vi "HFRR ADV v023 new software.vi"() -> ()   [LabVIEW 2025] (continued)
        n1928 = Divide(x=1705.984, y=w2075) -> (x/y=w2076:dbl)
        n1929 = Divide(x=1705.984, y=w2088) -> (x/y=w2089:dbl)
        n1930 = local read "Humidity before test"() -> (w2080:dbl)
        n1931 = local read "Humidity after test"() -> (w2093:dbl)
        n1932 = Subtract(x=8.017352 ("y"), y=w2076) -> (x-y=w2102:dbl)
        n1933 = Subtract(x=8.017352 ("y"), y=w2089) -> (x-y=w2096:dbl)
        n1934 = expression code="10**y"(w2102) -> (w2082:dbl)
        n1935 = expression code="10**y"(w2096) -> (w2095:dbl)
        n1936 = Multiply(x=w2080, y=w2082) -> (x*y=w2081:dbl)
        n1937 = Multiply(x=w2093, y=w2095) -> (x*y=w2094:dbl)
        n1938 = Divide(x=w2081, y=750.0) -> (x/y=w2097:dbl)
        n1939 = Divide(x=w2094, y=750.0) -> (x/y=w2098:dbl)
        n1940 = Add(x=w2097, y=w2098) -> (x+y=w2099:dbl)
        n1941 = Divide(x=w2099, y=2.0) -> (x/y=w2101:dbl)
        n1942 = local write "AVP"(w2101) -> ()
        n1943 = Subtract(x=1.4, y=w2101) -> (x-y=w2084:dbl)
        n1944 = local read "HCF"() -> (w2085:dbl)
      }
      frame Enabled {
      }
    }
    n1945 = case shown="True" "EDIT 3" {
      frame False {
      }
      frame True {
        n1946 = local write "EDIT 3"(FALSE ("EDIT 3")) -> ()
        n1947 = local write "Main Tab"(T2."About" ("Main Tab")) -> ()
      }
    }
    n1948 = case shown="False" w2070 {
      frame False {
        n1949 = local read "stopT"() -> (w3048:bool)
        n1950 = case shown="True" w3048 {
          frame False {
          }
          frame True {
            n1951 = local write "stopT"(FALSE) -> ()
          }
        }
      }
      frame True {
        "stopT" <- TRUE
      }
    }
    n1952 = case shown="False" w2068 {
      frame False {
      }
      frame True {
      }
    }
    n1953 = case shown="True" w2058 {
      frame False {
        n1954 = property on="Password 2" class="Str"("Visible"=FALSE) -> ()  [unwired: 2 in, 2 out]
        n1955 = local write "Password 2"("" ("Password")) -> ()
      }
      frame True {
        n1956 = property on="Password 2" class="Str"("Visible"=TRUE) -> ()  [unwired: 2 in, 2 out]
        n1957 = Equal?(x="Password 2", y="HFRR1234") -> (x = y?=w2190:bool)
        n1958 = case shown="True" w2190 {
          tunnel: "Password 2" -> [w2193 _]
          frame False {
            n1959 = String Length(string=w2193) -> (length=w2194:i32)
            n1960 = Greater Than 0?(x=w2194) -> (x > 0?=w2192:bool)
            n1961 = case shown="False" w2192 {
              frame False {
                n1962 = property on="Password 2" class="Str"("Caption.Text"="Password (Advance Setting)") -> ()  [unwired: 2 in, 2 out]
              }
              frame True {
                n1963 = property on="Password 2" class="Str"("Caption.Text"="Incorrect Password!") -> ()  [unwired: 2 in, 2 out]
              }
            }
          }
          frame True {
            n1964 = local write "EDIT 2"(FALSE ("EDIT 2")) -> ()
            n1965 = local write "Password 2"("" ("Password")) -> ()
            n1966 = local write "Main Tab"(T2."Advance" ("Main Tab")) -> ()
            n1967 = local write "Main Dashboard Buttons"(T1."Advance" ("Main Dashboard Buttons")) -> ()
          }
        }
      }
    }
    n1968 = case shown="True" "Prog Uno" {
      frame False {
      }
      frame True {
        n1969 = stacked-sequence {
          frame #0 {
            n1970 = Delete(path (use dialog)=path "C:/LAB-IQ-NXT/UNOCOMPILE.bat" ("working directory")) -> ()  [unwired: 4 in, 3 out]
          }
          frame #1 {
            n1971 = local read "Com Port 1"() -> (w2655:refnum<visa-resource-name>)
            n1972 = Concatenate Strings("cmd.exe /c \"mode " ("command line"), w2655, ":1200,n,8,1\"\n" ("command line")) -> (w2660:string)
            n1973 = Concatenate Strings(w2660, "CD\\\nCD WinDucom\navrdude -C avrdude.conf -v -patmega328p -carduino -P" ("command line"), w2655, " -b115200 -D -Uflash:w:UNO_V20.hex:i\n" ("command line"), "\r") -> (w2662:string)
            "STR" <- w2662
            n1974 = call <vilib>:"Write Characters To File.vi"("append to file? (new file:F)"=FALSE, "character string"=w2662, "file path (dialog if empty)"=path "C:/LAB-IQ/UNOCOMPILE.bat" ("working directory")) -> ()  [unwired: 2 in, 1 out]
          }
          frame #2 {
            n1975 = disable-structure shown="Disabled" {
              frame Disabled {
                w2666 = "cmd.exe  /c \"C:\\LAB-IQ-NXT\\UNOCOMPILE.bat\"" ("string")
                n1976 = local write "Prog Uno"(FALSE ("run minimized? (F)")) -> ()
                n1977 = call <vilib>:"System Exec.vi"("expected output size  (4096)"=u32 65535, "run minimized? (F)"=FALSE, "wait until completion? (T)"=TRUE ("run minimized? (F)"), "working directory"=path "C:/LAB-IQ-NXT", "standard input"=w2666, "command line"=w2666) -> ("error out"=w2665:errorcluster, "standard output"=→"String 42":string)  [unwired: 2 in, 2 out]
                "error out 3" <- w2665
                n1978 = flat-sequence {
                  tunnel: w2665 -> [_]
                  frame #0 {
                  }
                }
              }
              frame Enabled {
              }
            }
          }
        }
      }
    }
    n1979 = case shown="\"ISO 12156\"" "TEST STANDARD" {
      tunnel: [2.0 ("Set Temp") 0.0 ("Set Temp") 2.0 ("Set Temp") 0.0 ("Set Temp")] -> w2059
      frame "ASTM D6079", Default {
        w2612 = 50.0 ("Hz")
        w2613 = 53.0 ("Set Rh")
        w2615 = 1.0 ("Set Strk")
        w2614 = 60.0 ("Set Temp")
        # "astm hide"
        n1980 = local write "NORMAL LOAD"(200.0 ("NORMAL LOAD")) -> ()
        n1981 = local write "Set Strk"(w2615) -> ()
        n1982 = local write "Set Hz"(w2612) -> ()
        n1983 = local write "Set Temp"(w2614) -> ()
        n1984 = local write "Set Rh"(w2613) -> ()
        n1985 = local write "test time"(75.0 ("test time")) -> ()
        n1986 = local write "Set Stroke:"(w2615) -> ()
        n1987 = local write "Set Humidity:"(w2613) -> ()
        n1988 = local write "Set Frequency:"(w2612) -> ()
        n1989 = local write "Set Temperature:"(w2614) -> ()
        "Test Standard" <- "ASTM D6079" ("Test Standard 2")
      }
      frame "ISO 12156" {
        n1990 = local write "Set Strk"(1.0 ("Set Strk")) -> ()
        n1991 = local write "NORMAL LOAD"(200.0 ("NORMAL LOAD")) -> ()
        n1992 = local write "Set Temp"(60.0 ("Set Temp")) -> ()
        n1993 = local write "test time"(75.0 ("test time")) -> ()
        n1994 = local write "Set Hz"(50.0 ("Hz")) -> ()
        n1995 = local write "Set Rh"(53.0 ("Set Rh")) -> ()
      }
      frame "CEC F-096-A-06" {
        n1996 = local write "Set Strk"(1.0 ("Set Strk")) -> ()
        n1997 = local write "NORMAL LOAD"(200.0 ("NORMAL LOAD")) -> ()
        n1998 = local write "Set Temp"(60.0 ("Set Temp")) -> ()
        n1999 = local write "test time"(75.0 ("test time")) -> ()
        n2000 = local write "Set Hz"(50.0 ("Hz")) -> ()
        n2001 = local write "Set Rh"(53.0 ("Set Rh")) -> ()
      }
      frame "Custom" {
      }
    }
    n2002 = case shown="True" "Prog Due" {
      frame False {
      }
      frame True {
        n2003 = stacked-sequence {
          frame #0 {
            n2004 = Delete(path (use dialog)=path "C:/LAB-IQ/DUECOMPILE.bat" ("working directory")) -> ()  [unwired: 4 in, 3 out]
          }
          frame #1 {
            n2005 = disable-structure shown="Disabled" {
              frame Disabled {
                n2006 = local read "visa due"() -> (w2637:string)
                n2007 = Concatenate Strings("cmd.exe /c \"mode " ("command line"), w2637, ":1200,n,8,1\"\n" ("command line")) -> (w2642:string)
                n2008 = Concatenate Strings(w2642, "CD\\\nCD WinDucom\nTIMEOUT 1\n bossac.exe -i -d --port=" ("command line"), w2637, " -U false -e -w -v -b DUE.bin -R\n" ("command line"), "\r") -> (w2644:string)
                "concatenated string 2" <- w2644
                n2009 = call <vilib>:"Write Characters To File.vi"("append to file? (new file:F)"=FALSE, "character string"=w2644, "file path (dialog if empty)"=path "C:/LAB-IQ-NXT/DUECOMPILE.bat" ("working directory")) -> ()  [unwired: 2 in, 1 out]
              }
              frame Enabled {
              }
            }
          }
          frame #2 {
            # "C:\\LAB-IQ-NXT\\DUECOMPILE.bat"
            n2010 = disable-structure shown="Disabled" {
              frame Disabled {
                w2649 = "cmd.exe  /c \"C:\\LAB-IQ-NXT\\DUECOMPILE.bat\"" ("string")
                n2011 = call <vilib>:"System Exec.vi"("expected output size  (4096)"=u32 65535, "run minimized? (F)"=FALSE, "wait until completion? (T)"=TRUE ("run minimized? (F)"), "working directory"=path "C:/LAB-IQ-NXT", "standard input"=w2649, "command line"=w2649) -> ("error out"=w2648:errorcluster, "standard output"=→"String 44":string)  [unwired: 2 in, 2 out]
                "error out 4" <- w2648
                n2012 = flat-sequence {
                  tunnel: w2648 -> [_]
                  frame #0 {
                  }
                }
              }
              frame Enabled {
              }
            }
            n2013 = local write "Prog Due"(FALSE ("Prog Due")) -> ()
          }
        }
      }
    }
    n2014 = Or(x=w2056, y=w2054) -> (x .or. y?=w2055:bool)
    n2015 = case shown="\"About\"" w2053 {
      tunnel: [T27."Acquire" ("Main Tab") T27."Compare Files" ("Main Tab") T27."About" ("Main Tab")] -> w2066
      frame "Acquire", Default {
      }
      frame "Compare Files" {
      }
      frame "About" {
      }
    }
    n2016 = Or(x=w2060, y="OPEN") -> (x .or. y?=w2061:bool)
    n2017 = case shown="True" w2061 {
      tunnel: w2060 -> [_ w2201]
      frame False {
      }
      frame True {
        n2018 = stacked-sequence {
          tunnel: w2201 -> [_ w2268 _ _]
          frame #0 {
            w2217 = "  " ("String 6")
            n2019 = local write "OPEN"(FALSE ("open")) -> ()
            n2020 = local read "string1 2"() -> (w2205:string)
            n2021 = local read "string1 3"() -> (w2204:string)
            n2022 = local read "string1 4"() -> (w2203:string)
            n2023 = property on="OPEN" class="Bool (strict)"("Visible"=FALSE) -> ()  [unwired: 2 in, 2 out]
            n2024 = local write "String 6"(w2217) -> ()
            n2025 = local write "String 7"(w2217) -> ()
            n2026 = local write "String 8"(w2217) -> ()
            n2027 = local write "String 12"(w2217) -> ()
            n2028 = local read "OK Button 16"() -> (w2202:bool)
            n2029 = String To Path(string=w2205) -> (path=w2213:path)
            n2030 = String To Path(string=w2204) -> (path=w2212:path)
            n2031 = String To Path(string=w2203) -> (path=w2211:path)
            n2032 = case shown="True" w2202 {
              tunnel: [w2218 w2219] -> w2206
              frame False {
                n2033 = local read "string1"() -> (w2218:string)
              }
              frame True {
                n2034 = local read "String Indicator 4"() -> (w2219:string)
              }
            }
            n2035 = Open/Create/Replace File "Open File"(file path (use dialog)=w2213) -> (refnum out=w2209:refnum<file>)  [unwired: 5 in, 2 out]
            n2036 = Open/Create/Replace File "Open File"(file path (use dialog)=w2212) -> (refnum out=w2208:refnum<file>)  [unwired: 5 in, 2 out]
            n2037 = Open/Create/Replace File "Open File"(file path (use dialog)=w2211) -> (refnum out=w2207:refnum<file>)  [unwired: 5 in, 2 out]
            n2038 = while {
              tunnel: w2209 -> [w2231]
              i -> [w2227]
              stop <- w2226 continue-if-true
              (unwired) TRUE ("line mode (F)")
              n2039 = Read from Text File "Read File"(file (use dialog)=w2231) -> (text=w2228:string)  [unwired: 3 in, 3 out]
              n2040 = local write "Numeric 11"(w2227) -> ()
              n2041 = String Length(string=w2228) -> (length=w2230:i32)
              n2042 = Greater?(x=w2230, y=1) -> (0:w2226:bool)
            }
            n2043 = while {
              tunnel: w2208 -> [w2237]
              i -> [w2233]
              stop <- w2232 continue-if-true
              (unwired) TRUE ("line mode (F)")
              n2044 = Read from Text File "Read File"(file (use dialog)=w2237) -> (text=w2234:string)  [unwired: 3 in, 3 out]
              n2045 = local write "Numeric 12"(w2233) -> ()
              n2046 = String Length(string=w2234) -> (length=w2236:i32)
              n2047 = Greater?(x=w2236, y=1) -> (0:w2232:bool)
            }
            n2048 = while {
              tunnel: w2207 -> [w2243]
              i -> [w2239]
              stop <- w2238 continue-if-true
              (unwired) TRUE ("line mode (F)")
              n2049 = Read from Text File "Read File"(file (use dialog)=w2243) -> (text=w2240:string)  [unwired: 3 in, 3 out]
              n2050 = local write "Numeric 13"(w2239) -> ()
              n2051 = String Length(string=w2240) -> (length=w2242:i32)
              n2052 = Greater?(x=w2242, y=1) -> (0:w2238:bool)
            }
            n2053 = String To Path(string=w2206) -> (path=w2214:path)
            n2054 = Open/Create/Replace File "Open File"(file path (use dialog)=w2214) -> (refnum out=w2210:refnum<file>)  [unwired: 5 in, 2 out]
            n2055 = while {
              tunnel: w2210 -> [w2225]
              i -> [w2221]
              stop <- w2220 continue-if-true
              (unwired) TRUE ("line mode (F)")
              n2056 = Read from Text File "Read File"(file (use dialog)=w2225) -> (text=w2222:string)  [unwired: 3 in, 3 out]
              n2057 = local write "Numeric 8"(w2221) -> ()
              n2058 = String Length(string=w2222) -> (length=w2224:i32)
              n2059 = Greater?(x=w2224, y=1) -> (0:w2220:bool)
            }
          }
          frame #1 {
            w2395 = FALSE ("ACTUAL   MERGE")
            # "Sample Temp"
            # "ECR"
            # "COF"
            # "Time\nCOF\nFF\nTemp"
            n2060 = case shown="True" w2268 {
              tunnel: [w2415 w2416] -> w2269
              frame False {
                n2061 = local read "string1"() -> (w2415:string)
              }
              frame True {
                n2062 = local read "String Indicator 4"() -> (w2416:string)
              }
            }
            n2063 = local read "string1 3"() -> (w2313:string)
            n2064 = String To Path(string=w2269) -> (path=w2400:path)
            n2065 = String To Path(string=w2313) -> (path=w2411:path)
            n2066 = local read "Numeric 12"() -> (w2397:i32)
            n2067 = local read "Numeric 8"() -> (w2399:i32)
            n2068 = local read "string1 2"() -> (w2314:string)
            n2069 = local read "string1 4"() -> (w2312:string)
            n2070 = Open/Create/Replace File "Open File"(file path (use dialog)=w2400) -> (refnum out=w2414:refnum<file>, error out=w2413:errorcluster)  [unwired: 5 in, 1 out]
            n2071 = Open/Create/Replace File "Open File"(file path (use dialog)=w2411) -> (refnum out=w2407:refnum<file>, error out=w2408:errorcluster)  [unwired: 5 in, 1 out]
            n2072 = for {
              N: w2399 -> [_]
              tunnel: w2414 -> [w2562]
              tunnel: w2413 -> [w2561]
              tunnel: [w2551] -> w2326 mode=indexing
              tunnel: [w2549] -> w2383 mode=indexing
              tunnel: [w2550] -> w2378 mode=indexing
              tunnel: w2395 -> [_]
              tunnel: [w2543] -> w2380 mode=indexing
              tunnel: [w2539] -> w2349 mode=indexing
              tunnel: [w2535] -> w2324 mode=indexing
              tunnel: [w2531] -> w2305 mode=indexing
              tunnel: [w2526] -> w2265 mode=indexing
              (unwired) TRUE ("line mode (F)")
              # "freq"
              # "Stroke"
              # "Time"
              # "CoF"
              # "Humidity"
              # "Temp"
              # "Air Temp"
              # "ECR"
              n2073 = Read from Text File "Read File"(file (use dialog)=w2562, error in=w2561) -> (text=w2527:string)  [unwired: 2 in, 3 out]
              n2074 = local write "String 6"(w2527) -> ()
              n2075 = String Subset(string=w2527, offset (0)=0, length (rest)=14 ("length (rest)")) -> (substring=w2555:string)
              n2076 = String Subset(string=w2527, offset (0)=35, length (rest)=9 ("length (rest)")) -> (substring=w2552:string)
              n2077 = String Subset(string=w2527, offset (0)=15, length (rest)=9 ("length (rest)")) -> (substring=w2558:string)
              n2078 = Fract/Exp String To Number(string=w2555) -> (number=w2551:dbl)  [unwired: 3 in, 1 out]
              n2079 = Fract/Exp String To Number(string=w2552) -> (number=w2550:dbl)  [unwired: 3 in, 1 out]
              n2080 = Fract/Exp String To Number(string=w2558) -> (number=w2549:dbl)  [unwired: 3 in, 1 out]
              n2081 = String Subset(string=w2527, offset (0)=85, length (rest)=9 ("length (rest)")) -> (substring=w2528:string)
              n2082 = String Subset(string=w2527, offset (0)=25, length (rest)=9 ("length (rest)")) -> (substring=w2534:string)
              n2083 = String Subset(string=w2527, offset (0)=55, length (rest)=9 ("length (rest)")) -> (substring=w2536:string)
              n2084 = String Subset(string=w2527, offset (0)=45, length (rest)=9 ("length (rest)")) -> (substring=w2542:string)
              n2085 = String Subset(string=w2527, offset (0)=65, length (rest)=9 ("length (rest)")) -> (substring=w2548:string)
              n2086 = Fract/Exp String To Number(string=w2534) -> (number=w2531:dbl)  [unwired: 3 in, 1 out]
              n2087 = Fract/Exp String To Number(string=w2528) -> (number=w2526:dbl)  [unwired: 3 in, 1 out]
              n2088 = Fract/Exp String To Number(string=w2536) -> (number=w2535:dbl)  [unwired: 3 in, 1 out]
              n2089 = Fract/Exp String To Number(string=w2542) -> (number=w2539:dbl)  [unwired: 3 in, 1 out]
              n2090 = Fract/Exp String To Number(string=w2548) -> (number=w2545:dbl)  [unwired: 3 in, 1 out]
              n2091 = Add(x=w2545, y=0.0) -> (x+y=w2543:dbl)
            }
            n2092 = for {
              N: w2397 -> [_]
              tunnel: w2408 -> [w2488]
              tunnel: w2407 -> [w2487]
              tunnel: [w2477] -> w2366 mode=indexing
              tunnel: [w2475] -> w2364 mode=indexing
              tunnel: [w2476] -> w2360 mode=indexing
              tunnel: w2395 -> [_]
              tunnel: [w2469] -> w2362 mode=indexing
              tunnel: [w2465] -> w2344 mode=indexing
              tunnel: [w2461] -> w2320 mode=indexing
              tunnel: [w2458] -> w2301 mode=indexing
              tunnel: [w2454] -> w2260 mode=indexing
              (unwired) 9 ("length (rest)")
              (unwired) 9 ("length (rest)")
              (unwired) TRUE ("line mode (F)")
              n2093 = Read from Text File "Read File"(file (use dialog)=w2487, error in=w2488) -> (text=w2455:string)  [unwired: 2 in, 3 out]
              n2094 = local write "String 8"(w2455) -> ()
              n2095 = String Subset(string=w2455, offset (0)=85) -> (substring=w2457:string)  [unwired: 1 in]
              n2096 = String Subset(string=w2455, offset (0)=35, length (rest)=9 ("length (rest)")) -> (substring=w2478:string)
              n2097 = String Subset(string=w2455, offset (0)=55, length (rest)=9 ("length (rest)")) -> (substring=w2463:string)
              n2098 = String Subset(string=w2455, offset (0)=25) -> (substring=w2459:string)  [unwired: 1 in]
              n2099 = String Subset(string=w2455, offset (0)=15, length (rest)=9 ("length (rest)")) -> (substring=w2484:string)
              n2100 = String Subset(string=w2455, offset (0)=0, length (rest)=14 ("length (rest)")) -> (substring=w2481:string)
              n2101 = String Subset(string=w2455, offset (0)=45, length (rest)=9 ("length (rest)")) -> (substring=w2468:string)
              n2102 = String Subset(string=w2455, offset (0)=65, length (rest)=9 ("length (rest)")) -> (substring=w2474:string)
              n2103 = Fract/Exp String To Number(string=w2457) -> (number=w2454:dbl)  [unwired: 3 in, 1 out]
              n2104 = Fract/Exp String To Number(string=w2478) -> (number=w2476:dbl)  [unwired: 3 in, 1 out]
              n2105 = Fract/Exp String To Number(string=w2463) -> (number=w2461:dbl)  [unwired: 3 in, 1 out]
              n2106 = Fract/Exp String To Number(string=w2459) -> (number=w2458:dbl)  [unwired: 3 in, 1 out]
              n2107 = Fract/Exp String To Number(string=w2484) -> (number=w2475:dbl)  [unwired: 3 in, 1 out]
              n2108 = Fract/Exp String To Number(string=w2481) -> (number=w2477:dbl)  [unwired: 3 in, 1 out]
              n2109 = Fract/Exp String To Number(string=w2468) -> (number=w2465:dbl)  [unwired: 3 in, 1 out]
              n2110 = Fract/Exp String To Number(string=w2474) -> (number=w2471:dbl)  [unwired: 3 in, 1 out]
              n2111 = Add(x=w2471, y=0.0) -> (x+y=w2469:dbl)
            }
            n2112 = String To Path(string=w2314) -> (path=w2412:path)
            n2113 = String To Path(string=w2312) -> (path=w2406:path)
            n2114 = local read "Numeric 11"() -> (w2396:i32)
            n2115 = local read "Numeric 13"() -> (w2398:i32)
            n2116 = Open/Create/Replace File "Open File"(file path (use dialog)=w2412) -> (refnum out=w2410:refnum<file>, error out=w2409:errorcluster)  [unwired: 5 in, 1 out]
            n2117 = Open/Create/Replace File "Open File"(file path (use dialog)=w2406) -> (refnum out=w2405:refnum<file>, error out=w2404:errorcluster)  [unwired: 5 in, 1 out]
            n2118 = for {
              N: w2396 -> [_]
              tunnel: w2410 -> [w2525]
              tunnel: w2409 -> [w2524]
              tunnel: [w2514] -> w2376 mode=indexing
              tunnel: [w2512] -> w2374 mode=indexing
              tunnel: [w2513] -> w2369 mode=indexing
              tunnel: w2395 -> [_]
              tunnel: [w2506] -> w2371 mode=indexing
              tunnel: [w2502] -> w2347 mode=indexing
              tunnel: [w2498] -> w2322 mode=indexing
              tunnel: [w2494] -> w2303 mode=indexing
              tunnel: [w2489] -> w2261 mode=indexing
              (unwired) TRUE ("line mode (F)")
              n2119 = Read from Text File "Read File"(file (use dialog)=w2525, error in=w2524) -> (text=w2490:string)  [unwired: 2 in, 3 out]
              n2120 = local write "String 7"(w2490) -> ()
              n2121 = String Subset(string=w2490, offset (0)=85, length (rest)=9 ("length (rest)")) -> (substring=w2493:string)
              n2122 = String Subset(string=w2490, offset (0)=35, length (rest)=9 ("length (rest)")) -> (substring=w2515:string)
              n2123 = String Subset(string=w2490, offset (0)=55, length (rest)=9 ("length (rest)")) -> (substring=w2501:string)
              n2124 = String Subset(string=w2490, offset (0)=25, length (rest)=9 ("length (rest)")) -> (substring=w2495:string)
              n2125 = String Subset(string=w2490, offset (0)=45, length (rest)=9 ("length (rest)")) -> (substring=w2503:string)
              n2126 = String Subset(string=w2490, offset (0)=0, length (rest)=14 ("length (rest)")) -> (substring=w2518:string)
              n2127 = String Subset(string=w2490, offset (0)=15, length (rest)=9 ("length (rest)")) -> (substring=w2521:string)
              n2128 = String Subset(string=w2490, offset (0)=65, length (rest)=9 ("length (rest)")) -> (substring=w2507:string)
              n2129 = Fract/Exp String To Number(string=w2493) -> (number=w2489:dbl)  [unwired: 3 in, 1 out]
              n2130 = Fract/Exp String To Number(string=w2515) -> (number=w2513:dbl)  [unwired: 3 in, 1 out]
              n2131 = Fract/Exp String To Number(string=w2501) -> (number=w2498:dbl)  [unwired: 3 in, 1 out]
              n2132 = Fract/Exp String To Number(string=w2495) -> (number=w2494:dbl)  [unwired: 3 in, 1 out]
              n2133 = Fract/Exp String To Number(string=w2503) -> (number=w2502:dbl)  [unwired: 3 in, 1 out]
              n2134 = Fract/Exp String To Number(string=w2518) -> (number=w2514:dbl)  [unwired: 3 in, 1 out]
              n2135 = Fract/Exp String To Number(string=w2521) -> (number=w2512:dbl)  [unwired: 3 in, 1 out]
              n2136 = Fract/Exp String To Number(string=w2507) -> (number=w2510:dbl)  [unwired: 3 in, 1 out]
              n2137 = Add(x=w2510, y=0.0) -> (x+y=w2506:dbl)
            }
            n2138 = for {
              N: w2398 -> [_]
              tunnel: w2405 -> [w2453]
              tunnel: w2404 -> [w2452]
              tunnel: [w2442] -> w2358 mode=indexing
              tunnel: [w2441] -> w2351 mode=indexing
              tunnel: w2395 -> [_]
              tunnel: [w2430] -> w2356 mode=indexing
              tunnel: [w2435] -> w2353 mode=indexing
              tunnel: [w2431] -> w2343 mode=indexing
              tunnel: [w2426] -> w2318 mode=indexing
              tunnel: [w2422] -> w2299 mode=indexing
              tunnel: [w2417] -> w2259 mode=indexing
              (unwired) 1.0 ("x")
              (unwired) TRUE ("line mode (F)")
              n2139 = Read from Text File "Read File"(file (use dialog)=w2453, error in=w2452) -> (text=w2418:string)  [unwired: 2 in, 3 out]
              n2140 = local write "String 12"(w2418) -> ()
              n2141 = String Subset(string=w2418, offset (0)=85, length (rest)=9 ("length (rest)")) -> (substring=w2420:string)
              n2142 = String Subset(string=w2418, offset (0)=35, length (rest)=9 ("length (rest)")) -> (substring=w2443:string)
              n2143 = String Subset(string=w2418, offset (0)=55, length (rest)=9 ("length (rest)")) -> (substring=w2428:string)
              n2144 = String Subset(string=w2418, offset (0)=25, length (rest)=9 ("length (rest)")) -> (substring=w2424:string)
              n2145 = String Subset(string=w2418, offset (0)=45, length (rest)=9 ("length (rest)")) -> (substring=w2433:string)
              n2146 = String Subset(string=w2418, offset (0)=15, length (rest)=9 ("length (rest)")) -> (substring=w2449:string)
              n2147 = String Subset(string=w2418, offset (0)=0, length (rest)=14 ("length (rest)")) -> (substring=w2446:string)
              n2148 = String Subset(string=w2418, offset (0)=65, length (rest)=9 ("length (rest)")) -> (substring=w2436:string)
              n2149 = Fract/Exp String To Number(string=w2420) -> (number=w2417:dbl)  [unwired: 3 in, 1 out]
              n2150 = Fract/Exp String To Number(string=w2443) -> (number=w2441:dbl)  [unwired: 3 in, 1 out]
              n2151 = Fract/Exp String To Number(string=w2428) -> (number=w2426:dbl)  [unwired: 3 in, 1 out]
              n2152 = Fract/Exp String To Number(string=w2424) -> (number=w2422:dbl)  [unwired: 3 in, 1 out]
              n2153 = Fract/Exp String To Number(string=w2433) -> (number=w2431:dbl)  [unwired: 3 in, 1 out]
              n2154 = Fract/Exp String To Number(string=w2449) -> (number=w2430:dbl)  [unwired: 3 in, 1 out]
              n2155 = Fract/Exp String To Number(string=w2446) -> (number=w2442:dbl)  [unwired: 3 in, 1 out]
              n2156 = Fract/Exp String To Number(string=w2436) -> (number=w2439:dbl)  [unwired: 3 in, 1 out]
              n2157 = Add(x=w2439, y=0.0) -> (x+y=w2435:dbl)
            }
            n2158 = Delete From Array(array=w2301, index=0) -> (array with subset deleted=w2274:dbl[])  [unwired: 1 in, 1 out]
            n2159 = Delete From Array(array=w2364, index=0) -> (array with subset deleted=w2337:dbl[])  [unwired: 1 in, 1 out]
            n2160 = Delete From Array(array=w2344, index=0) -> (array with subset deleted=w2332:dbl[])  [unwired: 1 in, 1 out]
            n2161 = Delete From Array(array=w2362, index=0) -> (array with subset deleted=w2363:dbl[])  [unwired: 1 in, 1 out]
            n2162 = call-poly <vilib>:"Mean.vi"("X"=w2274) -> ("mean"=→"КОФ2 4":dbl)  [unwired: 1 out]
            n2163 = call-poly <vilib>:"Mean.vi"("X"=w2337) -> ("mean"=→"КОФ3":dbl)  [unwired: 1 out]
            n2164 = call-poly <vilib>:"Mean.vi"("X"=w2332) -> ("mean"=→"CP3":dbl)  [unwired: 1 out]
            n2165 = Delete From Array(array=w2326, index=0) -> (array with subset deleted=w2253:dbl[])  [unwired: 1 in, 1 out]
            n2166 = Delete From Array(array=w2265, index=0) -> (array with subset deleted=w2252:dbl[])  [unwired: 1 in, 1 out]
            n2167 = Delete From Array(array=w2305, index=0) -> (array with subset deleted=w2276:dbl[])  [unwired: 1 in, 1 out]
            n2168 = Delete From Array(array=w2383, index=0) -> (array with subset deleted=w2338:dbl[])  [unwired: 1 in, 1 out]
            n2169 = Delete From Array(array=w2349, index=0) -> (array with subset deleted=w2334:dbl[])  [unwired: 1 in, 1 out]
            "array w/ subset deleted" <- w2334
            n2170 = Delete From Array(array=w2380, index=0) -> (array with subset deleted=w2381:dbl[])  [unwired: 1 in, 1 out]
            n2171 = call-poly <vilib>:"Mean.vi"("X"=w2276) -> ("mean"=→"КОФ2 2":dbl)  [unwired: 1 out]
            n2172 = call-poly <vilib>:"Mean.vi"("X"=w2338) -> ("mean"=→"КОФ1":dbl)  [unwired: 1 out]
            n2173 = Bundle "Bundle"(w2253, w2252) -> (w2258:cluster{dbl[], dbl[]})  [unwired: 1 in]
            n2174 = Bundle "Bundle"(w2253, w2381) -> (w2245:cluster{dbl[], dbl[]})  [unwired: 1 in]
            n2175 = Delete From Array(array=w2260, index=0) -> (array with subset deleted=w2248:dbl[])  [unwired: 1 in, 1 out]
            n2176 = Delete From Array(array=w2261, index=0) -> (array with subset deleted=w2250:dbl[])  [unwired: 1 in, 1 out]
            n2177 = Delete From Array(array=w2371, index=0) -> (array with subset deleted=w2372:dbl[])  [unwired: 1 in, 1 out]
            n2178 = Delete From Array(array=w2259, index=0) -> (array with subset deleted=w2246:dbl[])  [unwired: 1 in, 1 out]
            n2179 = Delete From Array(array=w2353, index=0) -> (array with subset deleted=w2354:dbl[])  [unwired: 1 in, 1 out]
            n2180 = Delete From Array(array=w2378, index=0) -> (array with subset deleted=w2284:dbl[])  [unwired: 1 in, 1 out]
            n2181 = Delete From Array(array=w2324, index=0) -> (array with subset deleted=w2280:dbl[])  [unwired: 1 in, 1 out]
            n2182 = Delete From Array(array=w2360, index=0) -> (array with subset deleted=w2282:dbl[])  [unwired: 1 in, 1 out]
            n2183 = Delete From Array(array=w2320, index=0) -> (array with subset deleted=w2278:dbl[])  [unwired: 1 in, 1 out]
            n2184 = Delete From Array(array=w2369, index=0) -> (array with subset deleted=w2283:dbl[])  [unwired: 1 in, 1 out]
            n2185 = Delete From Array(array=w2322, index=0) -> (array with subset deleted=w2279:dbl[])  [unwired: 1 in, 1 out]
            n2186 = Delete From Array(array=w2303, index=0) -> (array with subset deleted=w2275:dbl[])  [unwired: 1 in, 1 out]
            n2187 = Delete From Array(array=w2347, index=0) -> (array with subset deleted=w2333:dbl[])  [unwired: 1 in, 1 out]
            n2188 = Delete From Array(array=w2374, index=0) -> (array with subset deleted=w2335:dbl[])  [unwired: 1 in, 1 out]
            n2189 = Delete From Array(array=w2351, index=0) -> (array with subset deleted=w2281:dbl[])  [unwired: 1 in, 1 out]
            n2190 = Delete From Array(array=w2318, index=0) -> (array with subset deleted=w2277:dbl[])  [unwired: 1 in, 1 out]
            n2191 = Delete From Array(array=w2299, index=0) -> (array with subset deleted=w2273:dbl[])  [unwired: 1 in, 1 out]
            n2192 = Delete From Array(array=w2343, index=0) -> (array with subset deleted=w2331:dbl[])  [unwired: 1 in, 1 out]
            n2193 = Delete From Array(array=w2356, index=0) -> (array with subset deleted=w2336:dbl[])  [unwired: 1 in, 1 out]
            n2194 = Delete From Array(array=w2366, index=0) -> (array with subset deleted=w2249:dbl[])  [unwired: 1 in, 1 out]
            n2195 = Delete From Array(array=w2376, index=0) -> (array with subset deleted=w2251:dbl[])  [unwired: 1 in, 1 out]
            n2196 = Delete From Array(array=w2358, index=0) -> (array with subset deleted=w2247:dbl[])  [unwired: 1 in, 1 out]
            n2197 = Bundle "Bundle"(w2253, w2284) -> (w2271:cluster{dbl[], dbl[]})  [unwired: 1 in]
            n2198 = Bundle "Bundle"(w2253, w2338) -> (w2272:cluster{dbl[], dbl[]})  [unwired: 1 in]
            n2199 = Bundle "Bundle"(w2284, w2280) -> (w2286:cluster{dbl[], dbl[]})  [unwired: 1 in]
            n2200 = Bundle "Bundle"(w2249, w2248) -> (w2256:cluster{dbl[], dbl[]})  [unwired: 1 in]
            n2201 = Bundle "Bundle"(w2282, w2278) -> (w2288:cluster{dbl[], dbl[]})  [unwired: 1 in]
            n2202 = Bundle "Bundle"(w2249, w2282) -> (w2392:cluster{dbl[], dbl[]})  [unwired: 1 in]
            n2203 = Bundle "Bundle"(w2249, w2278) -> (w2316:cluster{dbl[], dbl[]})  [unwired: 1 in]
            n2204 = Bundle "Bundle"(w2249, w2337) -> (w2402:cluster{dbl[], dbl[]})  [unwired: 1 in]
            n2205 = Bundle "Bundle"(w2249, w2332) -> (w2340:cluster{dbl[], dbl[]})  [unwired: 1 in]
            n2206 = Bundle "Bundle"(w2249, w2363) -> (w2387:cluster{dbl[], dbl[]})  [unwired: 1 in]
            n2207 = Bundle "Bundle"(w2283, w2279) -> (w2287:cluster{dbl[], dbl[]})  [unwired: 1 in]
            n2208 = Bundle "Bundle"(w2251, w2250) -> (w2257:cluster{dbl[], dbl[]})  [unwired: 1 in]
            n2209 = Bundle "Bundle"(w2251, w2283) -> (w2394:cluster{dbl[], dbl[]})  [unwired: 1 in]
            n2210 = Bundle "Bundle"(w2251, w2279) -> (w2317:cluster{dbl[], dbl[]})  [unwired: 1 in]
            n2211 = Bundle "Bundle"(w2251, w2333) -> (w2341:cluster{dbl[], dbl[]})  [unwired: 1 in]
            n2212 = Bundle "Bundle"(w2251, w2335) -> (w2403:cluster{dbl[], dbl[]})  [unwired: 1 in]
            n2213 = Bundle "Bundle"(w2251, w2372) -> (w2385:cluster{dbl[], dbl[]})  [unwired: 1 in]
            n2214 = Bundle "Bundle"(w2281, w2277) -> (w2289:cluster{dbl[], dbl[]})  [unwired: 1 in]
            n2215 = Bundle "Bundle"(w2247, w2246) -> (w2255:cluster{dbl[], dbl[]})  [unwired: 1 in]
            n2216 = Bundle "Bundle"(w2247, w2281) -> (w2393:cluster{dbl[], dbl[]})  [unwired: 1 in]
            n2217 = Bundle "Bundle"(w2247, w2277) -> (w2315:cluster{dbl[], dbl[]})  [unwired: 1 in]
            n2218 = Bundle "Bundle"(w2247, w2331) -> (w2339:cluster{dbl[], dbl[]})  [unwired: 1 in]
            n2219 = Bundle "Bundle"(w2247, w2336) -> (w2401:cluster{dbl[], dbl[]})  [unwired: 1 in]
            n2220 = Bundle "Bundle"(w2247, w2354) -> (w2386:cluster{dbl[], dbl[]})  [unwired: 1 in]
            n2221 = call-poly <vilib>:"Mean.vi"("X"=w2334) -> ("mean"=→"CP1":dbl)  [unwired: 1 out]
            n2222 = call-poly <vilib>:"Mean.vi"("X"=w2275) -> ("mean"=→"КОФ2 3":dbl)  [unwired: 1 out]
            n2223 = call-poly <vilib>:"Mean.vi"("X"=w2333) -> ("mean"=→"CP2":dbl)  [unwired: 1 out]
            n2224 = call-poly <vilib>:"Mean.vi"("X"=w2335) -> ("mean"=→"КОФ2":dbl)  [unwired: 1 out]
            n2225 = call-poly <vilib>:"Mean.vi"("X"=w2273) -> ("mean"=→"КОФ2 5":dbl)  [unwired: 1 out]
            n2226 = call-poly <vilib>:"Mean.vi"("X"=w2331) -> ("mean"=→"CP4":dbl)  [unwired: 1 out]
            n2227 = call-poly <vilib>:"Mean.vi"("X"=w2336) -> ("mean"=→"КОФ4":dbl)  [unwired: 1 out]
            n2228 = Bundle "Bundle"(w2253, w2280) -> (w2244:cluster{dbl[], dbl[]})  [unwired: 1 in]
            n2229 = Bundle "Bundle"(w2253, w2334) -> (w2267:cluster{dbl[], dbl[]})  [unwired: 1 in]
            n2230 = Build Array "Build Array"(w2244, w2267) -> (w2270:cluster{dbl[], dbl[]}[])
            "XY Graph 17" <- w2270
            n2231 = Build Array "Build Array"(w2258, w2257, w2256, w2255) -> (→"Frequency ( Hz )":cluster{dbl[], dbl[]}[])
            n2232 = Build Array "Build Array"(w2286, w2287, w2288, w2289) -> (→"Air Temp ( °C ) vs Humidity ( % RH )":cluster{dbl[], dbl[]}[])
            n2233 = Build Array "Build Array"(w2271, w2394, w2392, w2393) -> (→"Air Temperature  ( °C )":cluster{dbl[], dbl[]}[])
            n2234 = Build Array "Build Array"(w2244, w2317, w2316, w2315) -> (→"Humidity ( %RH )":cluster{dbl[], dbl[]}[])
            n2235 = Build Array "Build Array"(w2272, w2403, w2402, w2401) -> (→"Coefficient Of Friction":cluster{dbl[], dbl[]}[])
            n2236 = Build Array "Build Array"(w2267, w2341, w2340, w2339) -> (→"Sample Temperature ( °C )":cluster{dbl[], dbl[]}[])
            n2237 = Build Array "Build Array"(w2245, w2385, w2387, w2386) -> (→"XY Graph 13":cluster{dbl[], dbl[]}[])
            n2238 = Bundle "Bundle"(w2253, w2276) -> (w2298:cluster{dbl[], dbl[]})  [unwired: 1 in]
            n2239 = Bundle "Bundle"(w2249, w2274) -> (w2296:cluster{dbl[], dbl[]})  [unwired: 1 in]
            n2240 = Bundle "Bundle"(w2251, w2275) -> (w2297:cluster{dbl[], dbl[]})  [unwired: 1 in]
            n2241 = Bundle "Bundle"(w2247, w2273) -> (w2295:cluster{dbl[], dbl[]})  [unwired: 1 in]
            n2242 = Build Array "Build Array"(w2298, w2297, w2296, w2295) -> (→"Stroke ( mm )":cluster{dbl[], dbl[]}[])
            n2243 = local write "XY Graph 16"(w2270) -> ()
          }
          frame #2 {
          }
          frame #3 {
            n2244 = local write "Numeric 8"(0 ("Numeric 8")) -> ()
            n2245 = local write "Numeric 11"(0 ("Numeric 11")) -> ()
            n2246 = local write "Numeric 12"(0 ("Numeric 12")) -> ()
            n2247 = local write "Numeric 13"(0 ("Numeric 13")) -> ()
            n2248 = property on="OPEN" class="Bool (strict)"("Visible"=TRUE) -> ()  [unwired: 2 in, 2 out]
            n2249 = local read "String Control 2"() -> (w2570:string)
            n2250 = local read "String Control 4"() -> (w2569:string)
            n2251 = local read "String Control 6"() -> (w2568:string)
            n2252 = local read "String Control 8"() -> (w2567:string)
            n2253 = Match Pattern(string=w2570, regular expression="Samples / cycle :- ") -> (after substring=w2584:string)  [unwired: 1 in, 3 out]
            n2254 = Match Pattern(string=w2570, regular expression="Frequency :- ") -> (after substring=w2603:string)  [unwired: 1 in, 3 out]
            n2255 = Match Pattern(string=w2569, regular expression="Samples / cycle :- ") -> (after substring=w2580:string)  [unwired: 1 in, 3 out]
            n2256 = Match Pattern(string=w2569, regular expression="Frequency :- ") -> (after substring=w2598:string)  [unwired: 1 in, 3 out]
            n2257 = Match Pattern(string=w2568, regular expression="Samples / cycle :- ") -> (after substring=w2576:string)  [unwired: 1 in, 3 out]
            n2258 = Match Pattern(string=w2568, regular expression="Frequency :- ") -> (after substring=w2593:string)  [unwired: 1 in, 3 out]
            n2259 = Match Pattern(string=w2567, regular expression="Samples / cycle :- ") -> (after substring=w2572:string)  [unwired: 1 in, 3 out]
            n2260 = Match Pattern(string=w2567, regular expression="Frequency :- ") -> (after substring=w2588:string)  [unwired: 1 in, 3 out]
            n2261 = String Subset(string=w2584, length (rest)=6 ("length (rest)")) -> (substring=w2586:string)  [unwired: 1 in]
            n2262 = String Subset(string=w2603, length (rest)=9 ("length (rest)")) -> (substring=w2605:string)  [unwired: 1 in]
            n2263 = String Subset(string=w2580, length (rest)=6 ("length (rest)")) -> (substring=w2582:string)  [unwired: 1 in]
            n2264 = String Subset(string=w2598, length (rest)=9 ("length (rest)")) -> (substring=w2600:string)  [unwired: 1 in]
            n2265 = String Subset(string=w2576, length (rest)=6 ("length (rest)")) -> (substring=w2578:string)  [unwired: 1 in]
            n2266 = String Subset(string=w2593, length (rest)=9 ("length (rest)")) -> (substring=w2595:string)  [unwired: 1 in]
            n2267 = String Subset(string=w2572, length (rest)=6 ("length (rest)")) -> (substring=w2574:string)  [unwired: 1 in]
            n2268 = String Subset(string=w2588, length (rest)=9 ("length (rest)")) -> (substring=w2590:string)  [unwired: 1 in]
            n2269 = Fract/Exp String To Number(string=w2586) -> (number=w2566:dbl)  [unwired: 3 in, 1 out]
            n2270 = Fract/Exp String To Number(string=w2605) -> (number=w2606:dbl)  [unwired: 3 in, 1 out]
            n2271 = Fract/Exp String To Number(string=w2582) -> (number=w2565:dbl)  [unwired: 3 in, 1 out]
            n2272 = Fract/Exp String To Number(string=w2600) -> (number=w2601:dbl)  [unwired: 3 in, 1 out]
            n2273 = Fract/Exp String To Number(string=w2578) -> (number=w2564:dbl)  [unwired: 3 in, 1 out]
            n2274 = Fract/Exp String To Number(string=w2595) -> (number=w2596:dbl)  [unwired: 3 in, 1 out]
            n2275 = Fract/Exp String To Number(string=w2574) -> (number=w2563:dbl)  [unwired: 3 in, 1 out]
            n2276 = Fract/Exp String To Number(string=w2590) -> (number=w2591:dbl)  [unwired: 3 in, 1 out]
            n2277 = local write "sample1"(w2566) -> ()
            n2278 = local write "freq1"(w2606) -> ()
            n2279 = local write "sample2"(w2565) -> ()
            n2280 = local write "freq2"(w2601) -> ()
            n2281 = local write "sample3"(w2564) -> ()
            n2282 = local write "freq3"(w2596) -> ()
            n2283 = local write "sample4"(w2563) -> ()
            n2284 = local write "freq 4"(w2591) -> ()
          }
        }
      }
    }
    n2285 = case shown="True" w2055 {
      selector: w2055 -> [_ w2183]
      frame False {
      }
      frame True {
        n2286 = Not(x=w2183) -> (.not. x?=w2179:bool)
        n2287 = local write "service 3"(w2179) -> ()
        n2288 = local write "OPEN 6"(w2179) -> ()
        n2289 = call <vilib>:"System Exec.vi"("wait until completion? (T)"=TRUE, "command line"="C:\\LAB-IQ\\Scar View.exe") -> ("error out"=→"error out 5":errorcluster)  [unwired: 6 in, 3 out]
      }
    }
    n2290 = case shown="\"Acquire\", Default" w2066 {
      frame "Acquire", Default {
        w3079 = 0.2 ("y")
        w3084 = 1.0 ("y")
        w3085 = 0.8 ("y")
        # "Elapsed time\ncof\nstroke\nAir temp\nTemp\nHumidity"
        n2291 = disable-structure shown="Disabled" {
          frame Disabled {
            n2292 = local read "Flag"() -> (w3102:dbl)
            n2293 = local read "RUN"() -> (w3099:bool)
            n2294 = Not(x=w3099) -> (.not. x?=w3098:bool)
            n2295 = Equal?(x=w3102, y=10.0) -> (x = y?=w3100:bool)
            n2296 = And(x=w3100, y=w3098) -> (x .and. y?=w3097:bool)
            n2297 = case shown="True" w3097 {
              frame False {
              }
              frame True {
                w3103 = FALSE ("Heater Button")
                n2298 = local write "Humidity"(w3103) -> ()
                n2299 = local write "Heater Button"(w3103) -> ()
              }
            }
          }
          frame Enabled {
          }
        }
        n2300 = disable-structure shown="Disabled" {
          frame Disabled {
            n2301 = case shown="True" {
              selector: _ -> [_ _]
              frame False {
              }
              frame True {
                w3194 = TRUE ("Heater")
                n2302 = local write "Humidity"(w3194) -> ()
                n2303 = local write "Heater Button"(w3194) -> ()
                n2304 = local read "TEST STANDARD"() -> (w3197:T3)
                n2305 = local read "TEST STANDARD"() -> (w3192:T3)
                n2306 = Equal?(x=w3197, y=enum16{"ASTM D6079", "ISO 12156", "Custom"}."ISO 12156" ("Test Standard")) -> (x = y?=w3195:bool)
                n2307 = Equal?(x=w3192, y=enum16{"ASTM D6079", "ISO 12156", "Custom"}."ASTM D6079" ("Test Standard")) -> (x = y?=w3191:bool)
                n2308 = case shown="True" w3195 {
                  frame False {
                  }
                  frame True {
                    n2309 = local write "Heater"(TRUE ("Heater")) -> ()
                    n2310 = local write "airtempflg"(FALSE ("airtempflg")) -> ()
                  }
                }
                n2311 = case shown="True" w3191 {
                  frame False {
                  }
                  frame True {
                    n2312 = local write "Heater"(FALSE ("Heater")) -> ()
                    n2313 = local write "airtempflg"(TRUE ("airtempflg")) -> ()
                  }
                }
              }
            }
          }
          frame Enabled {
          }
        }
        n2314 = stacked-sequence {
          frame #0 {
            n2315 = case shown="True" "RST FF" {
              frame False {
              }
              frame True {
                w3260 = 0.0 ("X Scale.Range:Maximum")
                n2316 = property on="Frictional Force ( N )" class="WFChart (strict)"("XScale.Maximum"=600.0 ("X Scale.Range:Maximum"), "XScale.Minimum"=w3260, "YScale.Maximum"=10.0 ("Y Scale.Range:Maximum"), "YScale.Minimum"=w3260) -> ()  [unwired: 2 in, 2 out]
              }
            }
          }
          frame #1 {
            n2317 = case shown="True" "RST TEMP" {
              frame False {
              }
              frame True {
                n2318 = property on="Temperature ( Deg C )" class="WFChart (strict)"("XScale.Minimum"=0.0 ("X Scale.Range:Minimum"), "XScale.Maximum"=600.0 ("X Scale.Range:Maximum"), "YScale.Minimum"=0.0 ("Y Scale.Range:Minimum"), "YScale.Maximum"=100.0 ("Y Scale.Range:Maximum")) -> ()  [unwired: 2 in, 2 out]
              }
            }
          }
          frame #2 {
            n2319 = case shown="True" "RSTCOF" {
              frame False {
              }
              frame True {
                n2320 = property on="Coefficient of Friction" class="WFChart (strict)"("XScale.Minimum"=0.0 ("X Scale.Range:Minimum"), "XScale.Maximum"=600.0 ("X Scale.Range:Maximum"), "YScale.Maximum"=1.0 ("X Scale.Range:Minimum"), "YScale.Minimum"=0.0 ("X Scale.Range:Minimum")) -> ()  [unwired: 2 in, 2 out]
              }
            }
          }
          frame #3 {
            n2321 = case shown="True" "RSTCOF 2" {
              frame False {
              }
              frame True {
                (unwired) 100.0 ("Y Scale.Range:Maximum")
                (unwired) 0.0 ("Y Scale.Range:Minimum")
                (unwired) 600.0 ("X Scale.Range:Maximum")
                (unwired) 0.0 ("X Scale.Range:Minimum")
              }
            }
          }
          frame #4 {
            n2322 = case shown="True" "RSTCOF 3" {
              frame False {
              }
              frame True {
                n2323 = property on="Electrical Contact Resistance ( % )" class="WFChart (strict)"("XScale.Minimum"=0.0 ("X Scale.Range:Minimum"), "XScale.Maximum"=600.0 ("X Scale.Range:Maximum"), "YScale.Minimum"=0.0 ("Y Scale.Range:Minimum"), "YScale.Maximum"=100.0 ("Y Scale.Range:Maximum")) -> ()  [unwired: 2 in, 2 out]
              }
            }
          }
        }
        n2324 = disable-structure shown="Disabled" {
          frame Disabled {
            n2325 = case shown="True" {
              selector: _ -> [_ _]
              frame False {
              }
              frame True {
                n2326 = local read "zflag 2"() -> (w3161:dbl)
                n2327 = local read "yflag"() -> (w3163:dbl)
                n2328 = Equal?(x=w3163, y=2.0 ("tflag")) -> (x = y?=w3165:bool)
                n2329 = Equal?(x=w3161, y=3.0 ("tflag")) -> (x = y?=w3164:bool)
                n2330 = And(x=w3165, y=w3164) -> (x .and. y?=w3159:bool)
                n2331 = case shown="True" w3159 {
                  frame False {
                  }
                  frame True {
                    w3190 = 0.0 ("zflag")
                    n2332 = local write "zflag"(w3190) -> ()
                    n2333 = local write "zflag 2"(w3190) -> ()
                    n2334 = Delete(path (use dialog)=path "C:/LAB-IQ-NXT/WO 2449 TT.sig" ("file path (dialog if empty)")) -> (deleted path=w3189:path)  [unwired: 4 in, 2 out]
                    n2335 = Delete(path (use dialog)=path "C:/LAB-IQ-NXT/WO 2449 TRH.sig" ("file path (dialog if empty)")) -> (deleted path=w3184:path)  [unwired: 4 in, 2 out]
                    n2336 = local read "SEN.RUN HRS"() -> (w3176:dbl)
                    n2337 = local read "SENSOR TIME"() -> (w3174:dbl)
                    n2338 = call <vilib>:"compatOverwrite.vi"("overwrite (F)"=TRUE) -> ("overwrite?"=w3166:T30)
                    n2339 = call <vilib>:"compatOverwrite.vi"("overwrite (F)"=TRUE) -> ("overwrite?"=w3170:T30)
                    n2340 = local read "Total No. of Tests"() -> (w3177:dbl)
                    n2341 = Add(x=w3174, y=w3176) -> (x+y=w3175:dbl)
                    "SEN.RUN HRS" <- w3175
                    n2342 = Open/Create/Replace File(file path (use dialog)=w3189, operation (0:open)=w3166) -> (refnum out=w3167:refnum<file>, error out=w3168:errorcluster)  [unwired: 4 in, 1 out]
                    n2343 = Open/Create/Replace File(file path (use dialog)=w3184, operation (0:open)=w3170) -> (refnum out=w3171:refnum<file>, error out=w3172:errorcluster)  [unwired: 4 in, 1 out]
                    n2344 = Deny Access(4:w3168, 6:T28."deny none" ("deny mode (2)"), 7:w3167) -> (3:w3188:refnum<file>)  [unwired: 1 out]
                    n2345 = Deny Access(4:w3172, 6:T28."deny none" ("deny mode (2)"), 7:w3171) -> (3:w3180:refnum<file>)  [unwired: 1 out]
                    n2346 = Number To Decimal String(number=w3177) -> (decimal integer string=w3185:string)  [unwired: 1 in]
                    n2347 = Number To Decimal String(number=w3175) -> (decimal integer string=w3181:string)  [unwired: 1 in]
                    n2348 = Write to Binary File(file (use dialog)=w3188, data=w3185, 5:FALSE ("prepend array or string size? (T)")) -> ()  [unwired: 3 in, 3 out]
                    n2349 = Write to Binary File(file (use dialog)=w3180, data=w3181, 5:FALSE ("prepend array or string size? (T)")) -> ()  [unwired: 3 in, 3 out]
                  }
                }
              }
            }
          }
          frame Enabled {
          }
        }
        n2350 = local read "RUN"() -> (w3088:bool)
        n2351 = local read "run replace"() -> (w3092:bool)
        n2352 = local read "run replace"() -> (w3091:bool)
        n2353 = case shown="True" w3088 {
          frame False {
            n2354 = local write "run replace"(FALSE ("run replace")) -> ()
          }
          frame True {
            "run replace" <- TRUE ("run replace")
          }
        }
        n2355 = local read "RUN"() -> (w3096:bool)
        n2356 = local read "Set Temp"() -> (w3058:dbl)
        n2357 = local read "SetTemp"() -> (w3060:dbl)
        n2358 = case shown="False" w3096 {
          tunnel: [FALSE ("TEST RUNNING") TRUE ("TEST RUNNING")] -> w3095
          frame False {
            w3279 = 0.0 ("Flag")
            n2359 = local write "Elapsed time"(0.0 ("elapsedtime")) -> ()
            n2360 = local write "Time Remaining"(w3279) -> ()
            n2361 = local write "Flag"(w3279) -> ()
            n2362 = local write "Remaining Time"(w3279) -> ()
          }
          frame True {
            n2363 = local write "Flag"(10.0 ("Flag")) -> ()
          }
        }
        n2364 = case shown="False" w3092 {
          frame False {
            n2365 = local read "zflag"() -> (→"zflag 2":dbl)
            n2366 = local write "yflag"(2.0 ("tflag")) -> ()
            n2367 = local write "FLAG 4"(0.0 ("FLAG")) -> ()
          }
          frame True {
            n2368 = local write "yflag"(1.0 ("tflag")) -> ()
            n2369 = local write "zflag"(3.0 ("zflag")) -> ()
          }
        }
        n2370 = local read "acq 2"() -> (w3090:bool)
        n2371 = local read "AIR TEMP"() -> (w3053:dbl)
        n2372 = local read "Amb temp"() -> (w3057:dbl)
        n2373 = case shown="True" "Save & Continue" {
          frame False {
          }
          frame True {
            "acq 2" <- TRUE ("acq 2")
          }
        }
        n2374 = local read "Set Rh"() -> (w3059:dbl)
        n2375 = Add(x=w3060, y=w3085) -> (x+y=w3086:dbl)
        n2376 = Subtract(x=w3060, y=w3085) -> (x-y=w3087:dbl)
        n2377 = Add(x=w3058, y=w3079) -> (x+y=w3080:dbl)
        n2378 = Subtract(x=w3058, y=w3079) -> (x-y=w3081:dbl)
        n2379 = And(x=w3090, y=w3091) -> (x .and. y?=w3089:bool)
        n2380 = Greater Or Equal?(x=w3053, y=15.0) -> (x >= y?=w3054:bool)
        "powstat" <- w3054
        n2381 = local read "Humidity ( %RH )"() -> (w3056:dbl)
        n2382 = case shown="True" "Save & Continue" {
          frame False {
          }
          frame True {
            n2383 = while {
              tunnel: "0123456789abcdefghijklmnopqrstuvwxyzABCDEFGHIJKLMNOPQRSTUVWXYZ" ("string 2") -> [w3250]
              shift-right: [w3248] -> w3243
              shift-left: "" -> [w3247]
              i -> [w3257]
              stop <- w3256 stop-if-true
              n2384 = Random Number (0-1)() -> (number: 0 to 1=w3251:dbl)
              n2385 = Multiply(x=w3251, y=62.0) -> (x*y=w3253:dbl)
              n2386 = Decrement(x="Length") -> (x-1=w3246:i16)
              n2387 = To Word Integer(number=w3253) -> (16bit integer=w3254:i16)
              n2388 = String Subset(string=w3250, offset (0)=w3254, length (rest)=1 ("length (rest)")) -> (substring=w3249:string)
              n2389 = Greater Or Equal?(x=w3257, y=w3246) -> (x >= y?=w3256:bool)
              n2390 = Concatenate Strings(w3249, w3247) -> (w3248:string)
            }
            n2391 = local write "UUID"(w3243) -> ()
          }
        }
        n2392 = In Range and Coerce(upper limit=w3086, x=w3057, lower limit=w3087) -> (In Range?=w3076:bool)  [unwired: 1 out]
        n2393 = Add(x=w3059, y=w3084) -> (x+y=w3083:dbl)
        n2394 = Subtract(x=w3059, y=w3084) -> (x-y=w3082:dbl)
        n2395 = local read "TEMP"() -> (w3055:dbl)
        n2396 = case shown="True" "Save & Continue" {
          frame False {
          }
          frame True {
            n2397 = local read "Operator ID"() -> (w3574:string)
            n2398 = local read "FILE"() -> (w3580:string)
            n2399 = String Length(string=w3580) -> (length=w3578:i32)
            n2400 = String Length(string=w3574) -> (length=w3575:i32)
            n2401 = Greater?(x=w3578, y=0) -> (0:w3577:bool)
            n2402 = Greater?(x=w3575, y=0) -> (0:w3573:bool)
            n2403 = And(x=w3577, y=w3573) -> (x .and. y?=w3572:bool)
            n2404 = case shown="True" w3572 {
              frame False {
                n2405 = stacked-sequence {
                  frame #0 {
                    n2406 = One Button Dialog(message="Please Enter a File Name and Operator ID to save data !", button name ("OK")="Ok") -> ()  [unwired: 1 out]
                  }
                  frame #1 {
                    n2407 = local write "Save & Continue"(FALSE ("OK Button")) -> ()
                  }
                }
                n2408 = local write "Save & Continue"(FALSE ("OK Button")) -> ()
              }
              frame True {
                n2409 = stacked-sequence {
                  frame #0 {
                    n2410 = local read "FILE"() -> (w3586:string)
                    n2411 = call "file check.vi"("file name in"=w3586) -> ("file name out"=w3585:string)  [unwired: 9 in, 1 out]
                    n2412 = call <vilib>:"Application Directory.vi"() -> ("Application Directory"=w3596:path)
                    n2413 = Build Path(base path=w3596, name or relative path="data") -> (appended path=w3595:path)
                    n2414 = call <vilib>:"Trim Whitespace.vi"("string"=w3585) -> ("trimmed string"=w3593:string)  [unwired: 1 in]
                    n2415 = call <vilib>:"Trim Whitespace.vi"("string"=w3585) -> ("trimmed string"=w3594:string)  [unwired: 1 in]
                    n2416 = List Folder(path=w3595) -> (folder names=w3591:string[])  [unwired: 3 in, 3 out]
                    n2417 = Match Pattern(string=w3593, regular expression="_(") -> (before substring=w3590:string)  [unwired: 1 in, 3 out]
                    n2418 = for {
                      tunnel: w3591 -> [w3605] mode=indexing
                      tunnel: w3590 -> [w3603]
                      shift-right: [w3601] -> w3588
                      shift-left: bool[] [] -> [w3602]
                      n2419 = Match Pattern(string=w3605, regular expression="_(") -> (before substring=w3604:string)  [unwired: 1 in, 3 out]
                      n2420 = Equal?(x=w3604, y=w3603) -> (x = y?=w3600:bool)
                      n2421 = case shown="True" w3600 {
                        tunnel: w3600 -> [_ w3608]
                        tunnel: w3602 -> [w3607 w3610]
                        tunnel: [w3607 w3609] -> w3601
                        frame False {
                        }
                        frame True {
                          n2422 = Insert Into Array(array=w3610, new element=w3608) -> (w3609:bool[])  [unwired: 1 in]
                        }
                      }
                    }
                    n2423 = Equal?(x=w3591, y=w3590) -> (x = y?=w3599:bool[])
                    n2424 = Or Array Elements(Boolean array=w3599) -> (logical OR=w3598:bool)
                    n2425 = Array Size(array=w3588) -> (size(s)=w3587:i32)
                    n2426 = case shown="True" w3598 {
                      tunnel: w3594 -> [_ w3618]
                      tunnel: w3587 -> [_ w3611]
                      frame False {
                      }
                      frame True {
                        n2427 = Number To Decimal String(number=w3611) -> (decimal integer string=w3614:string)  [unwired: 1 in]
                        n2428 = Search/Split String(string=w3618, search string/char (-)="_(" ("regular expression")) -> (substring before match=w3616:string)  [unwired: 1 in, 2 out]
                        n2429 = Concatenate Strings(w3616, "_(" ("regular expression"), w3614, ")" ("regular expression")) -> (w3612:string)
                        n2430 = local write "FILE"(w3612) -> ()
                      }
                    }
                  }
                  frame #1 {
                    w3620 = 0.0
                    w3633 = cluster{"y":dbl, dbl, "y":dbl}[] [] ("History Data")
                    w3634 = FALSE ("Heater Button")
                    (unwired) ")!" ("string")
                    (unwired) ")" ("string")
                    w3632 = dbl[] [] ("History Data")
                    w3638 = "\r"
                    # "C:\\WinDucom\\Data\\"
                    # "C:\\LAB-IQ-NXT\\data"
                    n2431 = local write "Humidity ( %RH )"(w3620) -> ()
                    n2432 = local write "Frequency ( Hz )"(w3620) -> ()
                    n2433 = local write "Stroke 3"(w3620) -> ()
                    n2434 = local write "speedop"(0.0 ("PIDclk 2")) -> ()
                    n2435 = local write "Set Temp 2"(65.0 ("Set Temp 2")) -> ()
                    n2436 = local write "AIR TEMP"(w3620) -> ()
                    n2437 = local write "clk"(0.0 ("clk")) -> ()
                    n2438 = local write "Stroke 4"(w3620) -> ()
                    n2439 = local write "COF 2"(w3620) -> ()
                    n2440 = local write "TEMP"(w3620) -> ()
                    n2441 = local write "ecr 3"(w3620) -> ()
                    n2442 = local write "FF 3"(w3620) -> ()
                    n2443 = local write "FF 2"(w3620) -> ()
                    n2444 = property on="Humidity ( %RH )" class="WFChart (strict)"("History Data"=w3632) -> ()  [unwired: 2 in, 2 out]
                    n2445 = property on="Coefficient of Friction" class="WFChart (strict)"("History Data"=w3632) -> ()  [unwired: 2 in, 2 out]
                    n2446 = property on="Coefficient of Friction" class="WFChart (strict)"("History Data"=w3632) -> ()  [unwired: 2 in, 2 out]
                    n2447 = property on="Frictional Force ( N )" class="WFChart (strict)"("History Data"=w3632) -> ()  [unwired: 2 in, 2 out]
                    n2448 = property on="Electrical Contact Resistance ( % )" class="WFChart (strict)"("History Data"=w3632) -> ()  [unwired: 2 in, 2 out]
                    n2449 = property on="Electrical Contact Resistance ( % )" class="WFChart (strict)"("History Data"=w3632) -> ()  [unwired: 2 in, 2 out]
                    n2450 = property on="Temperature ( Deg C )" class="WFChart (strict)"("History Data"=w3632) -> ()  [unwired: 2 in, 2 out]
                    n2451 = property on="Frictional Force ( N )" class="WFChart (strict)"("History Data"=w3632) -> ()  [unwired: 2 in, 2 out]
                    n2452 = property on="Coefficient of Friction" class="WFChart (strict)"("History Data"=w3632) -> ()  [unwired: 2 in, 2 out]
                    n2453 = property on="Frictional Force ( N )" class="WFChart (strict)"("History Data"=w3632) -> ()  [unwired: 2 in, 2 out]
                    n2454 = property on="Electrical Contact Resistance ( % )" class="WFChart (strict)"("History Data"=w3632) -> ()  [unwired: 2 in, 2 out]
                    n2455 = property on="Temperature ( Deg C )" class="WFChart (strict)"("History Data"=w3632) -> ()  [unwired: 2 in, 2 out]
                    n2456 = property on="Humidity ( %RH )" class="WFChart (strict)"("History Data"=w3632) -> ()  [unwired: 2 in, 2 out]
                    n2457 = property on="Stroke ( mm )" class="WFChart (strict)"("History Data"=w3633) -> ()  [unwired: 2 in, 2 out]
                    n2458 = property on="Stroke ( mm )" class="WFChart (strict)"("History Data"=w3633) -> ()  [unwired: 2 in, 2 out]
                    n2459 = local write "Humidity"(w3634) -> ()
                    n2460 = local write "Heater Button"(w3634) -> ()
                    n2461 = local read "FILE"() -> (w3628:string)
                    n2462 = disable-structure shown="Enabled" {
                      disable-tunnel: [w3673 _] -> w3619
                      frame Enabled {
                        n2463 = local read "NORMAL LOAD"() -> (w3673:dbl)
                      }
                      frame Disabled {
                      }
                    }
                    n2464 = call "file check.vi"("file name in"=w3628) -> ("error out"=w3631:errorcluster, "file name out"=w3625:string)  [unwired: 9 in]
                    n2465 = call "FILE PATH CREATION.vi"("error in"=w3631, "FILE NAME :"=w3625) -> ("FILE OUT"=w3624:path)  [unwired: 8 in, 1 out]
                    n2466 = Concatenate Strings(w3625, ".dgf" ("Substring")) -> (w3630:string)
                    n2467 = Concatenate Strings(w3625, ".duf" ("Substring")) -> (w3626:string)
                    n2468 = Multiply(x=w3619, y=1.0) -> (x*y=w3652:dbl)
                    n2469 = Build Path(base path=w3624, name or relative path=w3630) -> (appended path=w3623:path)
